vi "Ekran Güncelle (SubVI).vi"(6 "Bulunan In":string, 7 "Aranan Kelime":string, 10 "Harf":string) -> (1 "Bulundu?":bool, 2 "Görüntü":string, 4 "Bululnan Out":string)   [LabVIEW 8.6]
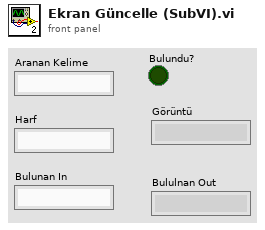
[diagram p1: front panel]
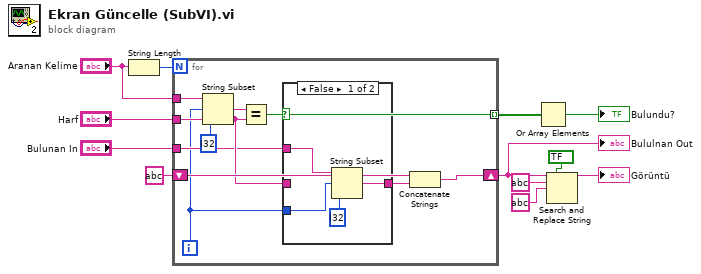
[diagram p0: block diagram]
diagram:
  n1 = String Length(string="Aranan Kelime") -> (length=w6:i32)
  n2 = for {
    N: w6 -> [_]
    tunnel: "Aranan Kelime" -> [w22]
    shift-right: [w18] -> w4
    shift-left: string ? ("BoolText.Text") -> [w19]
    tunnel: "Harf" -> [w17]
    tunnel: "Bulunan In" -> [w15]
    tunnel: [w13] -> w2 mode=indexing
    i -> [w14]
    n3 = String Subset(string=w22, offset (0)=w14, length (rest)=i32 ? ("length (rest)")) -> (substring=w20:string)
    n4 = Equal?(x=w20, y=w17) -> (x = y?=w13:bool)
    n5 = case shown="False" w13 {
      tunnel: w17 -> [_ w27]
      tunnel: [w25 w27] -> w16
      tunnel: w15 -> [w24 _]
      tunnel: w14 -> [w23 _]
      frame #0 {
        n6 = String Subset(string=w24, offset (0)=w23, length (rest)=i32 ? ("length (rest)")) -> (substring=w25:string)
      }
      frame #1 {
      }
    }
    n7 = Concatenate Strings(w19, w16) -> (w18:string)
  }
  "Bululnan Out" <- w4
  n8 = Or Array Elements(Boolean array=w2) -> (logical OR=→"Bulundu?":bool)
  n9 = Search and Replace String(replace all?=bool ? ("replace all? (F)"), input string=w4, search string=string ?, replace string=string ? ("replace string (\"\")")) -> (result string=→"Görüntü":string)  [unwired: 4 in, 3 out]
